vi "Apply Data To Tree.vi"(6 "Child Position":i32=-1, 8 "error in (no error)":errorcluster, 9 "Tree Item In":T1, 10 "Tree In":refnum<class "Tree.lvclass">, 11 "Tree Data in":refnum<class "Tree Data.lvclass">) -> (0 "error out":errorcluster, 2 "Tree Out":refnum<class "Tree.lvclass">, 3 "Tree Data out":refnum<class "Tree Data.lvclass">)   [LabVIEW 2024, in "Tree Data.lvclass"]
uses:
  Tree Data.lvclass
  Tree/Type Def/Tree Item.ctl
  Tree/Tree.lvclass
  Tree Data.lvclass/Tree Data.ctl
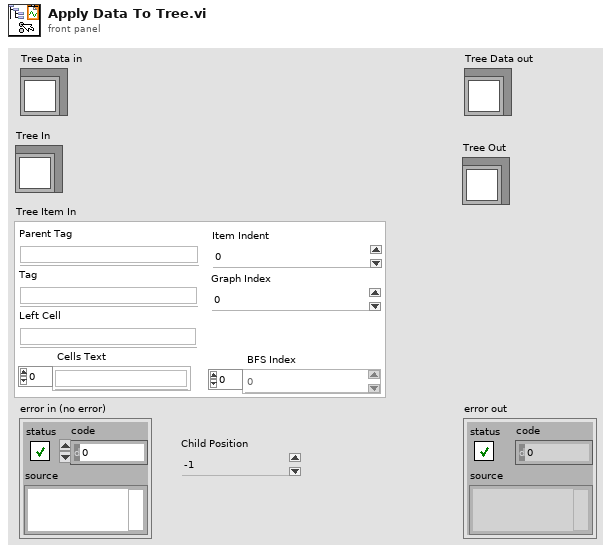
[diagram p1: front panel]
types:
  T1 = typedef "Tree Item.ctl" = cluster{"Parent Tag":string, "Tag":string, "Left Cell":string, "Cells Text":string[], "BFS Index":i32[], "Graph Index":i32, "Item Indent":i32}
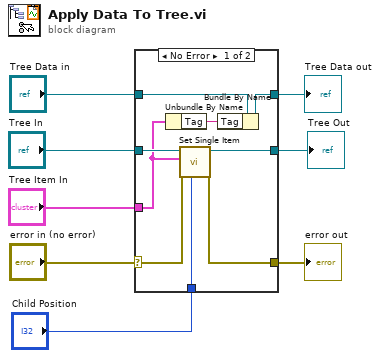
[diagram p0: block diagram]
diagram:
  n1 = case shown="No Error" "error in (no error)" {
    selector: "error in (no error)" -> [w15 w20]
    tunnel: [w14 w20] -> w7
    tunnel: [w12 w19] -> w5
    tunnel: "Tree Data in" -> [w13 w19]
    tunnel: "Tree Item In" -> [w11 _]
    tunnel: [w16 w18] -> w3
    tunnel: "Tree In" -> [w17 w18]
    tunnel: "Child Position" -> [w9 _]
    frame No Error {
      n2 = Unbundle By Name(w11) -> ("Tag"=w10:string)
      n3 = call "Set Single Item.vi"("Child Position"=w9, "error in (no error)"=w15, "Tree Item In"=w11, "Tree in"=w17) -> ("error out"=w14:errorcluster, "Tree out"=w16:refnum<class "Tree.lvclass">)  [unwired: 6 in]
      n4 = Bundle By Name(cluster=w13, "Tag"=w10) -> (w12:refnum<class "Tree Data.lvclass">)
    }
    frame Error {
    }
  }
  "error out" <- w7
  "Tree Data out" <- w5
  "Tree Out" <- w3
